vi "Get Direction.vi"(8 "error in (no error)":errorcluster, 11 "Impulse Manager in":refnum<class "Impulse Manager.lvclass">) -> (0 "error out":errorcluster, 2 "Direction":bool, 3 "Impulse Manager out":refnum<class "Impulse Manager.lvclass">)   [LabVIEW 2013, in "Impulse Manager.lvclass"]
uses:
  Impulse Manager.lvclass
  Impulse Manager.lvclass/Impulse Manager.ctl
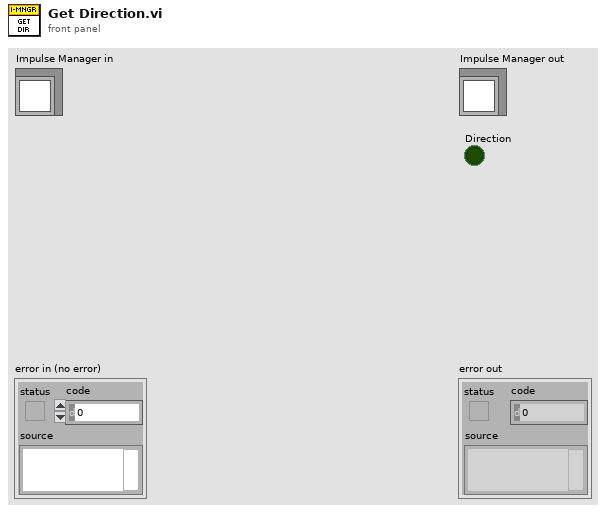
[diagram p1: front panel]
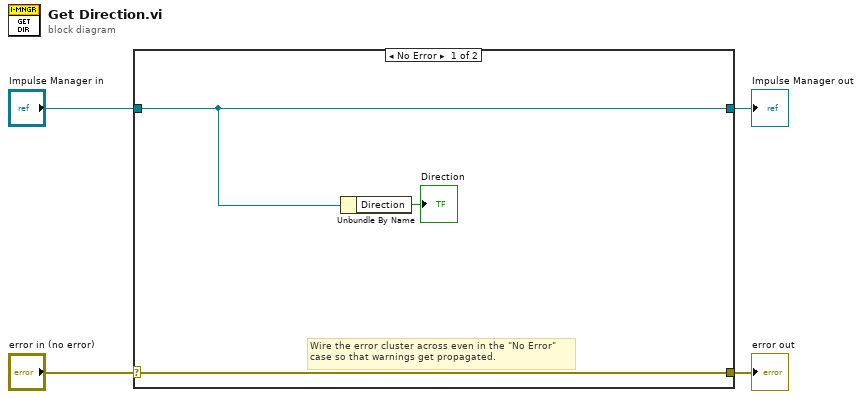
[diagram p0: block diagram]
diagram:
  n1 = case shown="No Error" "error in (no error)" {
    selector: "error in (no error)" -> [w7 w9]
    tunnel: [w7 w9] -> w3
    tunnel: [w6 w8] -> w1
    tunnel: "Impulse Manager in" -> [w6 w8]
    frame No Error {
      # "Wire the error cluster across even in the \"No Error\"\ncase so that warnings get propagated."
      n2 = Unbundle By Name(w6) -> ("Direction"=→"Direction":bool)
    }
    frame Error {
    }
  }
  "error out" <- w3
  "Impulse Manager out" <- w1
